vi "Ejercicio_10_initVariables.vi"() -> ()   [LabVIEW 2020]
panel:
  in  "stop":bool
  in  "Contraseña":string
  in  "Nombre":string
  out "Indicador contraseña":string
  out "Indicador nombre":string
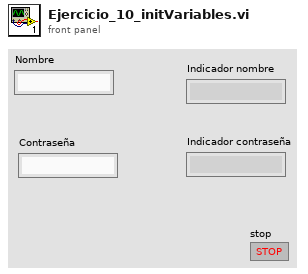
[diagram p1: front panel]
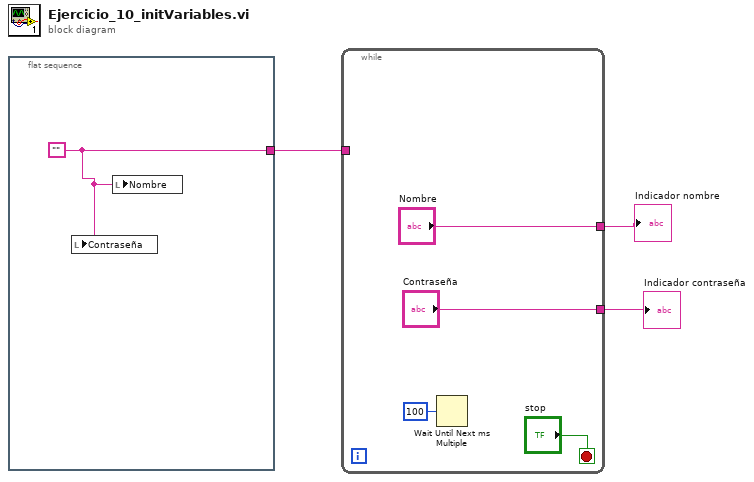
[diagram p0: block diagram]
diagram:
  n1 = flat-sequence {
    tunnel: [w4] -> w1
    frame #0 {
      w4 = ""
      n2 = local write "Contraseña"(w4) -> ()
      n3 = local write "Nombre"(w4) -> ()
    }
  }
  n4 = while {
    tunnel: ["Nombre"] -> w3
    tunnel: ["Contraseña"] -> w2
    tunnel: w1 -> [_]
    stop <- "stop" stop-if-true
    n5 = Wait Until Next ms Multiple(millisecond multiple=u32 100) -> ()  [unwired: 1 out]
  }
  "Indicador nombre" <- w3
  "Indicador contraseña" <- w2
